vi "myFinalProject.vi"() -> ()   [LabVIEW 2016]
panel:
  in  "Tab Control":enum32{"Page 1", " Add noise and filter"}(tab)
  in  "Path":path
  in  "JPEG/PNG":bool
  out "Red":u8[][](graph)
  out "Green":u8[][](graph)
  out "Blue":u8[][](graph)
  out "new picture":picture
  out "Blue original":u8[][](graph)
  out "Green original":u8[][](graph)
  out "Red original":u8[][](graph)
  out "Green Channel Added Noises":u8[][](graph)
  out "Blue Channel Added Noises":u8[][](graph)
  in  "Radio Buttons":T1(radio)
  in  "Choose Noise":string(combo)
  in  "Deviation":dbl=1.0000000000000002 format="%0.2f"
  in  "Seed":i32=-1
  in  "Amplifier":dbl=1.0000000000000002 format="%0.2f"
  out "Red Channel  Added Noises":u8[][](graph)
  out "Blue Filtered":dbl[][](graph)
  out "Green Filtered":dbl[][](graph)
  out "Red Filtered":dbl[][](graph)
  in  "Filters":T2(radio)
  in  "Filters 2":T2(radio)
  in  "Filters 3":T2(radio)
  in  "Filters 4":T2(radio)
  out "Run time costed":string
  out "Red Filtered Difference":dbl
  out "Green Filtered Difference":dbl
  out "Blue  Filtered Difference":dbl
  out "Red Noise Difference":dbl
  out "Green Noise Difference":dbl
  out "Blue  Noise Difference":dbl
  out "All Filtered Difference":dbl
  in  "Choose a path to store the difference value":path
  out "Original picture":picture
  out "new picture 3":picture
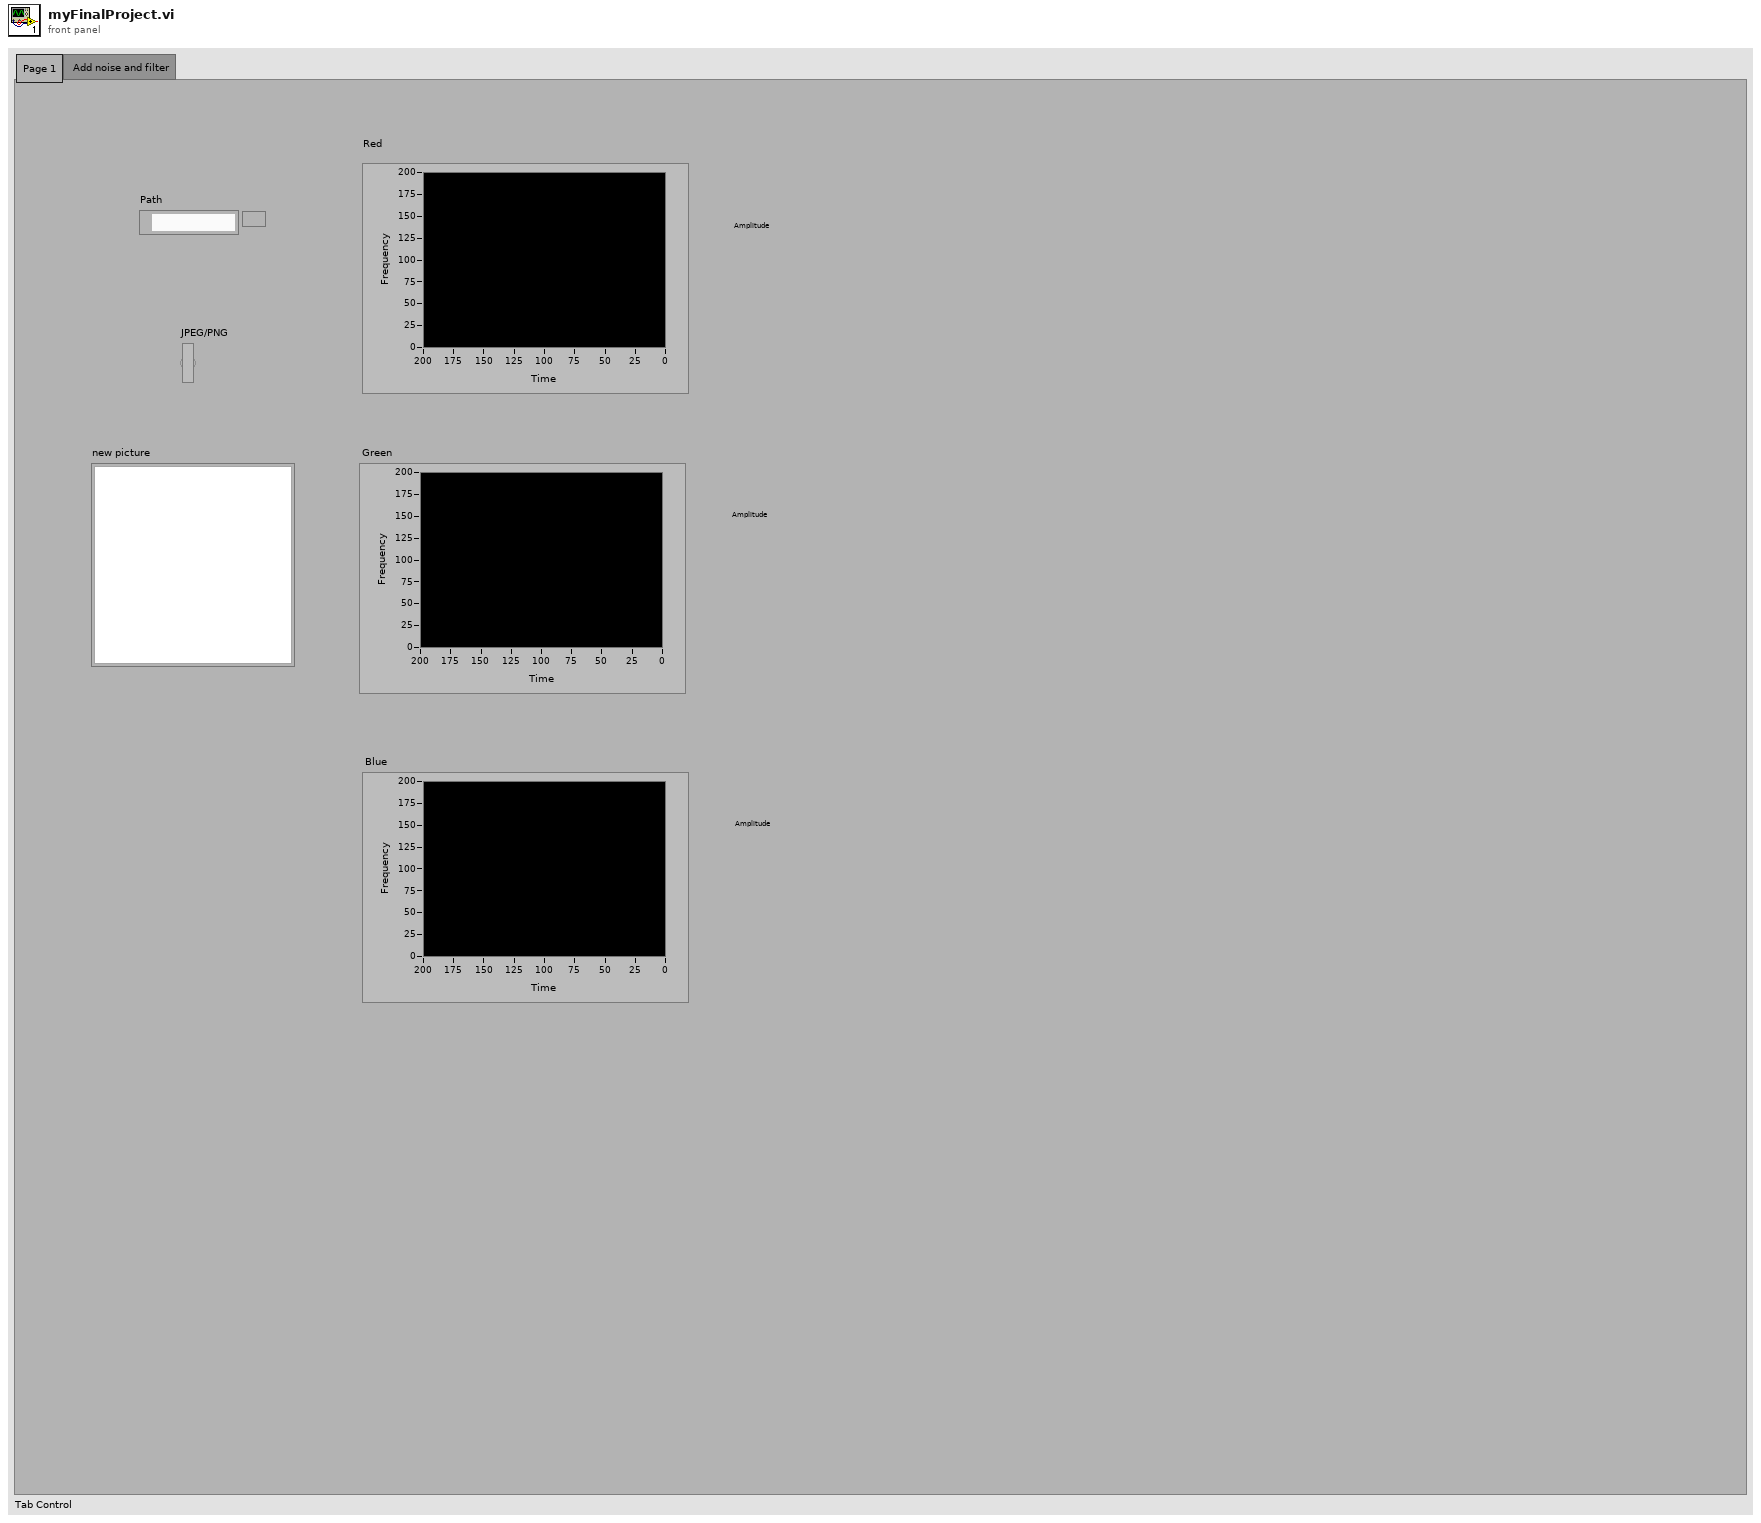
[diagram p1: front panel]
types:
  T1 = enum32{" Red Channel", "Green Channel", "Blue Channel", " All Channel"}
  T2 = enum32{"Lowpass ", "Highpass", "Band pass", "Band Stop", "Butter Worth ", "No filter"}
  T3 = typedef "imagedata.ctl" = cluster{"image type":i32, "image depth":i32, "image":u8[], "mask":u8[], "colors":u32[], "Rectangle":cluster{"left":i16, "top":i16, "right":i16, "bottom":i16}}
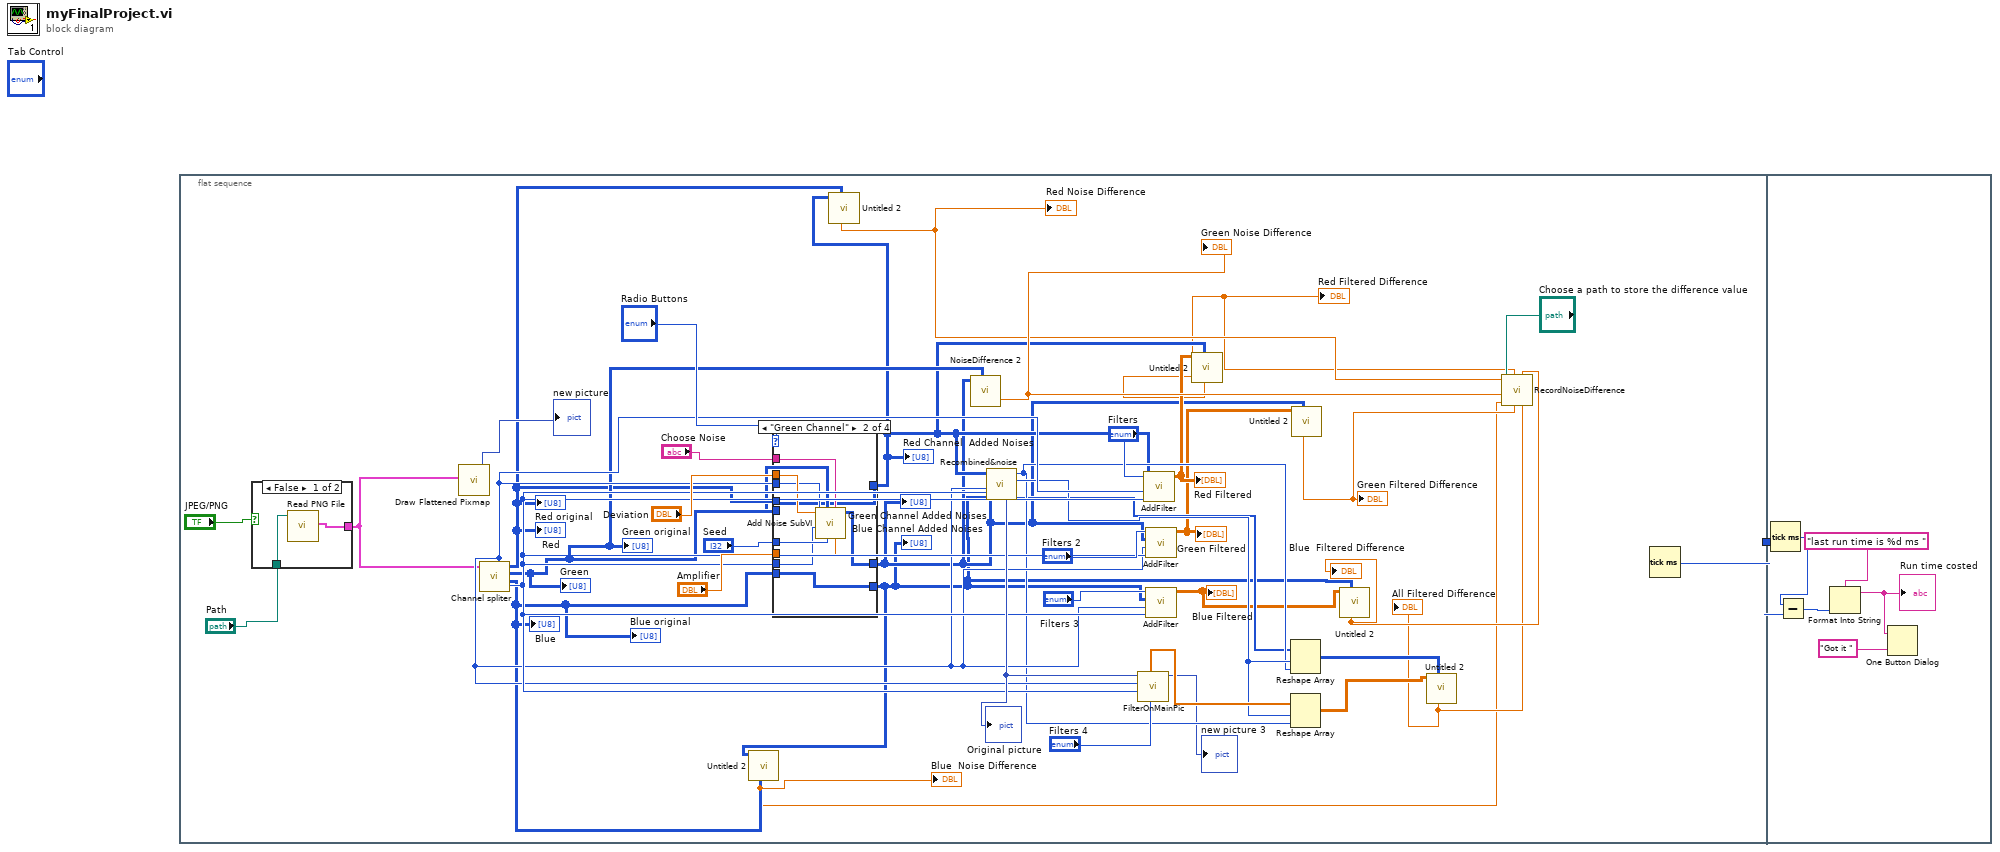
[diagram p0: block diagram]
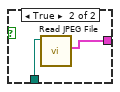
[diagram p2: hidden frame]
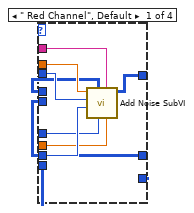
[diagram p3: hidden frame]
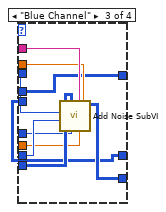
[diagram p4: hidden frame]
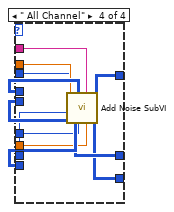
[diagram p5: hidden frame]
diagram:
  n1 = flat-sequence {
    tunnel: [w29] -> w1
    tunnel: w1 -> [w93]
    frame #0 {
      n2 = case shown="False" "JPEG/PNG" {
        tunnel: [w43 w45] -> w27
        tunnel: "Path" -> [w44 w46]
        frame False {
          n3 = call <vilib>:"Read PNG File.vi"("path to PNG file"=w44) -> ("image data"=w43:T3)  [unwired: 8 in, 2 out]
        }
        frame True {
          n4 = call <vilib>:"Read JPEG File.vi"("path to JPEG file"=w46) -> ("image data"=w45:T3)  [unwired: 8 in, 2 out]
        }
      }
      n5 = call <vilib>:"Draw Flattened Pixmap.vi"("image data"=w27) -> ("new picture"=→"new picture":picture)  [unwired: 8 in]
      n6 = call "Channel spliter.vi"("image data"=w27) -> ("Array 2"=w5:u8[][], "Array"=w19:u8[][], "Array 3"=w18:u8[][], "right"=w32:i16, "bottom"=w31:i16)  [unwired: 6 in]
      "Blue" <- w5
      "Green" <- w19
      "Red" <- w18
      "Red original" <- w18
      "Green original" <- w19
      "Blue original" <- w5
      n7 = case shown="\"Green Channel\"" "Radio Buttons" {
        tunnel: "Seed" -> [w53 w66 w71 w81]
        tunnel: "Amplifier" -> [w52 w65 w70 w80]
        tunnel: "Deviation" -> [w56 w64 w74 w84]
        tunnel: "Choose Noise" -> [w50 w63 w76 w85]
        tunnel: w31 -> [w55 w62 w73 w83]
        tunnel: w32 -> [w54 w61 w72 w82]
        tunnel: w19 -> [w47 w60 w68 w87]
        tunnel: w18 -> [w51 w58 w67 w88]
        tunnel: w5 -> [w48 w57 w75 w86]
        tunnel: [w49 w58 w67 w79] -> w16
        tunnel: [w47 w59 w68 w78] -> w13
        tunnel: [w48 w57 w69 w77] -> w4
        frame " Red Channel", Default {
          n8 = call "Add Noise SubVI.vi"("Noise Amplitude"=w52, "Choose Noise"=w50, "seed"=w53, "Input 1"=w51, "right"=w54, "bottom"=w55, "deviation"=w56) -> ("Output 1"=w49:u8[][])  [unwired: 2 in, 2 out]
        }
        frame "Green Channel" {
          n9 = call "Add Noise SubVI.vi"("Noise Amplitude"=w65, "Choose Noise"=w63, "seed"=w66, "Input 1"=w60, "right"=w61, "bottom"=w62, "deviation"=w64) -> ("Output 1"=w59:u8[][])  [unwired: 2 in, 2 out]
        }
        frame "Blue Channel" {
          n10 = call "Add Noise SubVI.vi"("Noise Amplitude"=w70, "Choose Noise"=w76, "seed"=w71, "Input 1"=w75, "right"=w72, "bottom"=w73, "deviation"=w74) -> ("Output 1"=w69:u8[][])  [unwired: 2 in, 2 out]
        }
        frame " All Channel" {
          n11 = call "Add Noise SubVI.vi"("Input 3"=w86, "Noise Amplitude"=w80, "Choose Noise"=w85, "seed"=w81, "Input 1"=w88, "Input 2"=w87, "right"=w82, "bottom"=w83, "deviation"=w84) -> ("Output 3"=w77:u8[][], "Output 2"=w78:u8[][], "Output 1"=w79:u8[][])
        }
      }
      "Red Channel  Added Noises" <- w16
      "Green Channel Added Noises" <- w13
      "Blue Channel Added Noises" <- w4
      n12 = call "Untitled 2.vi"("Before"=w5, "After"=w4) -> ("Numeric"=w3:dbl)  [unwired: 9 in]
      "Blue  Noise Difference" <- w3
      n13 = call "Untitled 2.vi"("Before"=w18, "After"=w16) -> ("Numeric"=w17:dbl)  [unwired: 9 in]
      "Red Noise Difference" <- w17
      n14 = call "NoiseDifference 2.vi"("Before"=w19, "After"=w13) -> ("Numeric"=w20:dbl)  [unwired: 9 in]
      "Green Noise Difference" <- w20
      n15 = call "Recombined&noise.vi"("right"=w32, "Input 3"=w4, "bottom"=w31, "input 2"=w13, "Inpupt"=w16) -> ("Rectangle.right"=w24:i16, "Rectangle.bottom"=w23:i16, "new picture"=w33:picture, "output image array"=w22:u8[])  [unwired: 3 in]
      "Original picture" <- w33
      n16 = call "FilterOnMainPic.vi"("Filters 4"="Filters 4", "right"=w32, "bottom"=w31, "Noised picture"=w33) -> ("Noise+Pic 2"=→"new picture 3":picture, "Filtered X"=w25:dbl[])  [unwired: 6 in]
      n17 = call "AddFilter.vi"("Bottom"=w32, "Right"=w31, "Output 1"=w16, "Filters"="Filters") -> ("Filtered X"=w15:dbl[][])  [unwired: 7 in]
      "Red Filtered" <- w15
      n18 = call "AddFilter.vi"("Bottom"=w32, "Right"=w31, "Output 1"=w13, "Filters"="Filters 2") -> ("Filtered X"=w12:dbl[][])  [unwired: 7 in]
      "Green Filtered" <- w12
      n19 = call "AddFilter.vi"("Bottom"=w32, "Right"=w31, "Output 1"=w4, "Filters"="Filters 3") -> ("Filtered X"=w10:dbl[][])  [unwired: 7 in]
      "Blue Filtered" <- w10
      n20 = call "Untitled 2.vi"("Before"=w16, "After"=w15) -> ("Numeric"=w14:dbl)  [unwired: 9 in]
      "Red Filtered Difference" <- w14
      n21 = Reshape Array(w22, w24, w23) -> (w8:u8[][])
      n22 = Reshape Array(w25, w24, w23) -> (w7:dbl[][])
      n23 = call "Untitled 2.vi"("Before"=w13, "After"=w12) -> ("Numeric"=w11:dbl)  [unwired: 9 in]
      "Green Filtered Difference" <- w11
      n24 = call "Untitled 2.vi"("Before"=w4, "After"=w10) -> ("Numeric"=w9:dbl)  [unwired: 9 in]
      "Blue  Filtered Difference" <- w9
      n25 = call "Untitled 2.vi"("Before"=w8, "After"=w7) -> ("Numeric"=w6:dbl)  [unwired: 9 in]
      "All Filtered Difference" <- w6
      n26 = call "RecordNoiseDifference.vi"("All f"=w6, "Blue f"=w9, "Green  f"=w11, "Red f"=w14, "Blue"=w3, "Green"=w20, "file path (use dialog)"="Choose a path to store the difference value", "Red"=w17) -> ()  [unwired: 4 in]
      n27 = Tick Count (ms)() -> (millisecond timer value=w29:u32)
    }
    frame #1 {
      n28 = Tick Count (ms)() -> (millisecond timer value=w94:u32)
      n29 = Subtract(x=w94, y=w93) -> (x-y=w92:u32)
      n30 = Format Into String(format string="last run time is %d ms " ("message"), w92) -> (resulting string=w90:string)  [unwired: 2 in, 1 out]
      "Run time costed" <- w90
      n31 = One Button Dialog(message=w90, button name ("OK")="Got it " ("message")) -> ()  [unwired: 1 out]
    }
  }
